vi "Async.Initialize.vi"(8 "error in (no error)":errorcluster, 9 "Processes":cluster{"VI":refnum<vi>, "Parameters":variant}[](array[cluster]), 10 "Name":string, 11 "Async in":refnum<class "VS Inline Async API.lvclass">) -> (0 "error out":errorcluster, 3 "Async out":refnum<class "VS Inline Async API.lvclass">)   [LabVIEW 2015, in "VS Inline Async API.lvlib" / "VS Inline Async API.lvclass"]
uses:
  VS Inline Async API.lvclass
  VS Inline Async API.lvclass/VS Inline Async API.ctl
  <vilib>/Utility/error.llb/Error Cluster From Error Code.vi
  VS Inline Async API.lvlib
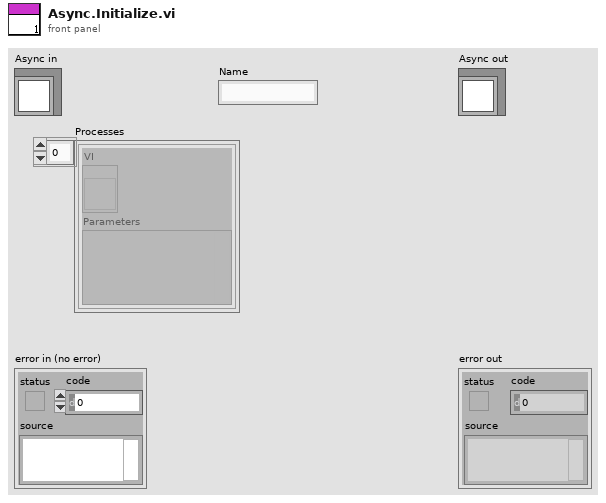
[diagram p1: front panel]
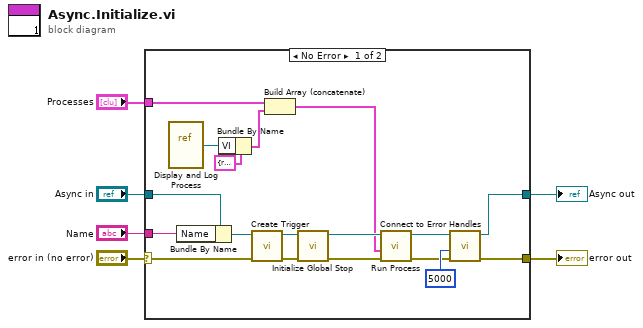
[diagram p0: block diagram]
diagram:
  n1 = case shown="No Error" "error in (no error)" {
    selector: "error in (no error)" -> [w23 w26]
    tunnel: [w15 w26] -> w5
    tunnel: [w13 w25] -> w3
    tunnel: "Async in" -> [w21 w25]
    tunnel: "Name" -> [w19 _]
    tunnel: "Processes" -> [w20 _]
    frame No Error {
      n2 = vi-ref "Display and Log Process.vi"() -> (w11:refnum<vi>)
      n3 = Bundle By Name(cluster=w21, "Name"=w19) -> (w22:refnum<class "VS Inline Async API.lvclass">)
      n4 = Bundle By Name(cluster=cluster{"VI":refnum<vi>, "Parameters":variant} {"VI"=refnum, "Parameters"=variant} ("Process"), "VI"=w11) -> (w10:cluster{"VI":refnum<vi>, "Parameters":variant})
      n5 = call "Create Trigger.vi"("error in (no error)"=w23, "Async in"=w22) -> ("error out"=w18:errorcluster, "Async out"=w17:refnum<class "VS Inline Async API.lvclass">)  [unwired: 8 in]
      n6 = Build Array (concatenate)(w20, w10) -> (w7:cluster{"VI":refnum<vi>, "Parameters":variant}[])
      n7 = call "Initialize Global Stop.vi"("error in (no error)"=w18, "Async in"=w17) -> ("error out"=w9:errorcluster, "Async out"=w8:refnum<class "VS Inline Async API.lvclass">)  [unwired: 8 in]
      n8 = call "Run Process.vi"("error in (no error)"=w9, "Processes"=w7, "Async in"=w8) -> ("error out"=w16:errorcluster, "Async out"=w14:refnum<class "VS Inline Async API.lvclass">)  [unwired: 7 in]
      n9 = call "Connect to Error Handles.vi"("error in"=w16, "Timeout (ms)"=u16 5000, "Async in"=w14) -> ("error out"=w15:errorcluster, "Async out"=w13:refnum<class "VS Inline Async API.lvclass">)  [unwired: 7 in]
    }
    frame Error {
    }
  }
  "error out" <- w5
  "Async out" <- w3
